vi "Robot_movimiento_calibración_NoLeeQR.vi"() -> ()   [LabVIEW 2019]
uses:
  <vilib>/Instr/_visa.llb/VISA Configure Serial Port (Instr).vi
  Global_STOP.vi
  <vilib>/regexp/Match Regular Expression.xnode
panel:
  in  "Bandeja Salida":bool=TRUE
  in  "stop socket 3":bool
  in  "stop 6":bool
  in  "Abrir socket 2":bool
  in  "Cerrar socket 2":bool
  in  "Interruptor Error 2":bool
  in  "stop 5":bool
  in  "STOP TEST 3":bool
  in  "Interruptor Error":bool
  in  "Cerrar socket":bool
  in  "Abrir socket":bool
  out "return count":u32
  out "lectura puerto serie":u32
  out "dato escrito puerto serie":string
  out "TEST OK":bool
  out "error out":errorcluster {"code" format="%f"}
  in  "STOP TEST 2":bool
  in  "SELECCION DE TEST":string(combo)="COMPLETO"
  in  "?":bool
  out "Boolean":bool
  in  "stop socket 2":bool
  out "Bytes at port 3":u32=1
  in  "IN y":string(combo)="00"
  in  "IN x":string(combo)="00"
  in  "NOK y":string(combo)="00"
  in  "NOK x":string(combo)="00"
  in  "OK y":string(combo)="00"
  in  "OK x":string(combo)="00"
  in  "Operator's name":string(combo)="Juan Rodríguez"
  in  "?":bool
  in  "Fichero de registro":path=path "C:/Trabajo_Robot/Pruebas/Pruebas.txt"
  in  "Path Out Report":path=path "C:/Trabajo_Robot/desde Marzo 2023/Pruebas_PC_APD/RESULT_TEST_C_LABP0/Test_33_ASIC_Referencia"
  in  "stop socket":bool
  out "Bytes at port 1":u32
  out "Iteraciones":i32
  out "Lectura buffer":string="1"
  in  "Delay (ms).Velocidad desplazamiento robot\nSi ponemos por ej. 2ms el robot va a la mitad de velocidad":dbl=1.0 min=1.0 max=9.0 step=1.0
  out "Bytes at port 2":u32=1
  in  "Interruptor":bool=TRUE
  in  "stop":bool
  # "SI SE PRESIONA EL BOTON STOP PARA INTERRUMPIR EL TEST,\nHAY QUE APAGAR Y VOLVER A ENCENDER EL ARDUINO\nCON EL SWITCH DE LA CAJA."
  # "TRUE : BANDEJA OK\nFALSE BANDEJA NOK"
  # "x: columna en cada bandeja \ny: fila en cada bandeja"
  # "Funcionamiento: en la primera iteración, el efector se desplaza desde el origen hasta la celda\nintroducida, hace una pausa, va a la posición del socket (0,0), hace otra pausa, va a la celda\nde salida y vuelve al origen. En las iteraciones siguientes hará lo mismo pero recorriendo las\nceldas de la bandeja sucesivamente. Que el desplazamiento se produzca hacia una celda de\nla bandeja OK o de la bandeja NOK depende de la salidad del programa de test de Asics."
types:
  T1 = enum16{"open", "replace", "create", "open or create", "replace or create", "replace or create with confirmation"}
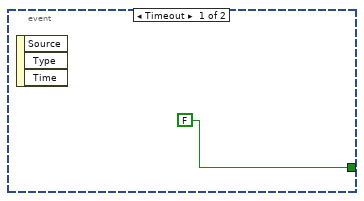
[diagram p2: hidden frame]
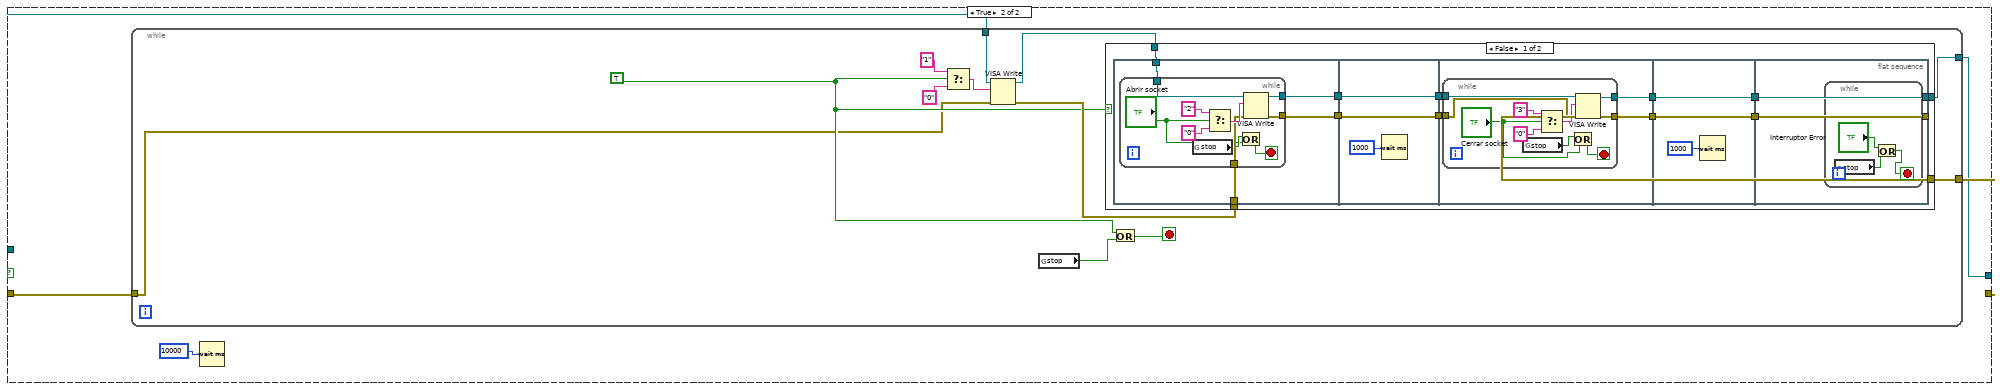
[diagram p3: hidden frame]
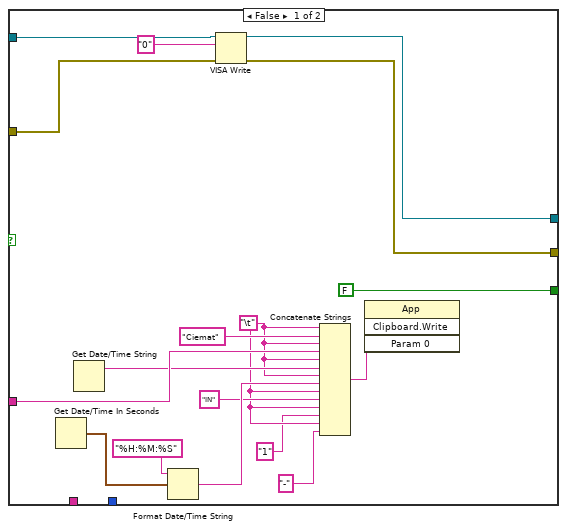
[diagram p5: hidden frame]
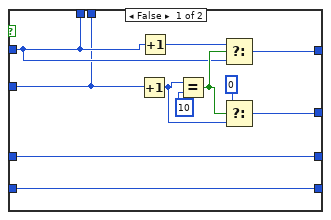
[diagram p7: hidden frame]
diagram:
  n1 = control-ref of="stop socket"() -> (w2:refnum<vi>)
  n2 = control-ref of="Cerrar socket"() -> (w10:refnum<vi>)
  n3 = control-ref of="STOP TEST 2"() -> (w13:refnum<vi>)
  n4 = control-ref of="Abrir socket"() -> (w8:refnum<vi>)
  n5 = control-ref of="stop"() -> (w9:refnum<vi>)
  n6 = control-ref of="Interruptor Error"() -> (w11:refnum<vi>)
  n7 = property class="Bool (strict)"(reference=w13, "Visible"=FALSE) -> ()  [unwired: 1 in, 2 out]
  n8 = property class="Bool"("Visible"=TRUE) -> ()  [unwired: 2 in, 2 out]
  n9 = property class="Bool (strict)"(reference=w8, "Visible"=FALSE) -> ()  [unwired: 1 in, 2 out]
  n10 = property class="Bool (strict)"(reference=w11, "Visible"=FALSE) -> ()  [unwired: 1 in, 2 out]
  n11 = property class="Bool (strict)"(reference=w10, "Visible"=FALSE) -> ()  [unwired: 1 in, 2 out]
  n12 = property on="Boolean" class="Bool (strict)"("Visible"=FALSE) -> ()  [unwired: 2 in, 2 out]
  n13 = property class="Bool"(reference=w2, "Visible"=FALSE) -> ()  [unwired: 1 in, 2 out]
  n14 = property class="Bool"(reference=w9, "Visible"=FALSE) -> ()  [unwired: 1 in, 2 out]
  n15 = flat-sequence {
    tunnel: [w56] -> w19
    tunnel: ["Fichero de registro"] -> w18
    tunnel: ["SELECCION DE TEST"] -> w17
    tunnel: ["NOK y"] -> w34
    tunnel: ["NOK x"] -> w33
    tunnel: ["OK y"] -> w32
    tunnel: ["OK x"] -> w31
    tunnel: ["IN y"] -> w30
    tunnel: ["IN x"] -> w29
    tunnel: [w59] -> w28
    tunnel: [w60] -> w27
    tunnel: ["IN y"] -> w26
    tunnel: ["IN x"] -> w25
    tunnel: w18 -> [w58]
    frame #0 {
      n16 = while {
        stop <- "?" stop-if-true
        n17 = Not(x="?") -> (.not. x?=w51:bool)
        "Boolean" <- w51
        n18 = property on="Boolean" class="Bool (strict)"("Blinking"=w51) -> ()  [unwired: 2 in, 2 out]
      }
      n19 = global write "Global_STOP.vi" "stop"(FALSE ("stop")) -> ()
    }
    frame #1 {
      n20 = property class="Bool"("Visible"=FALSE) -> ()  [unwired: 2 in, 2 out]
      n21 = Not(x="?") -> (.not. x?=w56:bool)
    }
    frame #2 {
      n22 = Open/Create/Replace File(file path (use dialog)=w58, operation (0:open)=T1."open", access (0:read/write)=enum16{"read/write", "read-only", "write-only"}."write-only") -> (refnum out=w71:refnum<file>, error out=w73:errorcluster)  [unwired: 3 in, 1 out]
      n23 = Set File Position(refnum=w71, from (0:start)=enum16{"start", "end", "current"}."end", error in=w73) -> (refnum out=w72:refnum<file>, error out=w74:errorcluster)  [unwired: 1 in]
      n24 = Write to Text File(file (use dialog)=w72, text="\r\n", error in=w74) -> (refnum out=w60:refnum<file>, error out=w59:errorcluster)  [unwired: 1 in, 1 out]
    }
  }
  n25 = Decimal String To Number(string=w26) -> (number=w24:i32)  [unwired: 2 in, 1 out]
  n26 = Decimal String To Number(string=w25) -> (number=w21:i32)  [unwired: 2 in, 1 out]
  n27 = Multiply(x=10, y=w24) -> (x*y=w22:i32)
  n28 = Decimal String To Number(string=w32) -> (number=w36:i32)  [unwired: 2 in, 1 out]
  n29 = Decimal String To Number(string=w31) -> (number=w35:i32)  [unwired: 2 in, 1 out]
  n30 = Decimal String To Number(string=w34) -> (number=w38:i32)  [unwired: 2 in, 1 out]
  n31 = Decimal String To Number(string=w33) -> (number=w37:i32)  [unwired: 2 in, 1 out]
  n32 = call-poly "VISA Configure Serial Port"("VISA resource name"=refnum<visa-resource-name> "COM9", "baud rate (9600)"=u32 9600, "data bits (8)"=u16 8) -> ("VISA resource name out"=w42:refnum<visa-resource-name>, "error out"=w45:errorcluster)  [unwired: 11 in]
  n33 = Add(x=w22, y=w21) -> (x+y=w20:i32)
  n34 = while {
    shift-right: [w75] -> w43
    shift-left: w45 -> [w116]
    tunnel: w42 -> [w114]
    tunnel: [w78] -> w44
    tunnel: w27 -> [w107]
    tunnel: [w106] -> w41
    tunnel: w28 -> [w105]
    tunnel: [w104] -> w40
    tunnel: w29 -> [w102]
    tunnel: w30 -> [w101]
    tunnel: w31 -> [w100]
    tunnel: w32 -> [w99]
    tunnel: w33 -> [w98]
    tunnel: w34 -> [w97]
    shift-right: [w90] -> _
    shift-left: w38 -> [w96]
    shift-right: [w92] -> _
    shift-left: w37 -> [w95]
    shift-right: [w89] -> _
    shift-left: w36 -> [w94]
    shift-right: [w91] -> _
    shift-left: w35 -> [w93]
    tunnel: w20 -> [w88]
    tunnel: w19 -> [w81]
    tunnel: w17 -> [w80]
    tunnel: [w77] -> w15
    i -> [w79]
    stop <- w77 stop-if-true
    # "Cuando Arduino deja un ASIC en la bandeja de  entrada ó en las de OK/NOK\ny vuelve a la posicion de socket, envia un \"2\" por el puerto serie\na labview y éste lo lee para que se salga del bucle, y prosiga la secuencia que le queda\nal programa, para después coger otro asic. Javier Morales"
    n35 = flat-sequence {
      tunnel: w116 -> [w154]
      tunnel: w114 -> [w143]
      tunnel: [w145] -> w113
      tunnel: [w144] -> w112
      tunnel: w102 -> [w124]
      tunnel: w101 -> [w123]
      tunnel: w100 -> [w122]
      tunnel: w99 -> [w121]
      tunnel: w98 -> [w120]
      tunnel: w97 -> [w119]
      tunnel: w113 -> [w891]
      tunnel: w112 -> [w890]
      tunnel: [w889] -> w87
      tunnel: [w888] -> w85
      tunnel: [w887] -> _
      tunnel: w87 -> [w908]
      tunnel: [w906] -> w86
      tunnel: w85 -> [w907]
      tunnel: [w905] -> w84
      tunnel: w86 -> [w928]
      tunnel: w84 -> [w927]
      tunnel: w79 -> [w929]
      tunnel: [w925] -> w83
      tunnel: [w924] -> w82
      tunnel: w79 -> [w1015]
      tunnel: [w1017] -> w110
      tunnel: [w1016] -> w109
      tunnel: [w1013] -> w103
      tunnel: w83 -> [w1012]
      tunnel: w82 -> [w1011]
      tunnel: w81 -> [w1006]
      tunnel: w80 -> [w1009]
      tunnel: w79 -> [w1008]
      tunnel: [w1065] -> w108
      tunnel: [w1067] -> w111
      tunnel: w110 -> [w1066]
      tunnel: w109 -> [w1064]
      tunnel: w107 -> [w1071]
      tunnel: [w1070] -> w106
      tunnel: w105 -> [w1069]
      tunnel: [w1068] -> w104
      tunnel: w79 -> [w1061]
      tunnel: w103 -> [w1060]
      tunnel: w96 -> [w1056]
      tunnel: w95 -> [w1059]
      tunnel: w94 -> [w1058]
      tunnel: w93 -> [w1057]
      tunnel: [w1055] -> w90
      tunnel: [w1054] -> w92
      tunnel: [w1053] -> w89
      tunnel: [w1052] -> w91
      tunnel: w88 -> [w1051]
      tunnel: w79 -> [w1050]
      tunnel: [w1049] -> _
      frame #0 {
        n36 = for {
          N: 2 -> [_]
          shift-right: [w766] -> _
          shift-left: w124 -> [w771]
          shift-right: [w769] -> w140
          shift-left: w143 -> [w770]
          shift-right: [w767] -> w139
          shift-left: w154 -> [w768]
          n37 = xnode "Match Regular Expression"("input string"=w771, "regular expression"="-?\\d") -> ("whole match"=w765:string, "after match"=w766:string)  [unwired: 4 in, 3 out]
          n38 = VISA Write(VISA resource name=w770, write buffer=w765, error in (no error)=w768) -> (VISA resource name out=w769:refnum<visa-resource-name>, error out=w767:errorcluster)  [unwired: 1 out]
        }
        n39 = for {
          N: 2 -> [_]
          shift-right: [w644] -> _
          shift-left: w123 -> [w649]
          shift-right: [w647] -> w134
          shift-left: w140 -> [w648]
          shift-right: [w645] -> w133
          shift-left: w139 -> [w646]
          n40 = xnode "Match Regular Expression"("input string"=w649, "regular expression"="-?\\d") -> ("whole match"=w643:string, "after match"=w644:string)  [unwired: 4 in, 3 out]
          n41 = VISA Write(VISA resource name=w648, write buffer=w643, error in (no error)=w646) -> (VISA resource name out=w647:refnum<visa-resource-name>, error out=w645:errorcluster)  [unwired: 1 out]
        }
        n42 = for {
          N: 2 -> [_]
          shift-right: [w522] -> _
          shift-left: w122 -> [w527]
          shift-right: [w525] -> w136
          shift-left: w134 -> [w526]
          shift-right: [w523] -> w135
          shift-left: w133 -> [w524]
          n43 = xnode "Match Regular Expression"("input string"=w527, "regular expression"="-?\\d") -> ("whole match"=w521:string, "after match"=w522:string)  [unwired: 4 in, 3 out]
          n44 = VISA Write(VISA resource name=w526, write buffer=w521, error in (no error)=w524) -> (VISA resource name out=w525:refnum<visa-resource-name>, error out=w523:errorcluster)  [unwired: 1 out]
        }
        n45 = for {
          N: 2 -> [_]
          shift-right: [w400] -> _
          shift-left: w121 -> [w405]
          shift-right: [w403] -> w128
          shift-left: w136 -> [w404]
          shift-right: [w401] -> w127
          shift-left: w135 -> [w402]
          n46 = xnode "Match Regular Expression"("input string"=w405, "regular expression"="-?\\d") -> ("whole match"=w399:string, "after match"=w400:string)  [unwired: 4 in, 3 out]
          n47 = VISA Write(VISA resource name=w404, write buffer=w399, error in (no error)=w402) -> (VISA resource name out=w403:refnum<visa-resource-name>, error out=w401:errorcluster)  [unwired: 1 out]
        }
        n48 = for {
          N: 2 -> [_]
          shift-right: [w278] -> _
          shift-left: w120 -> [w283]
          shift-right: [w281] -> w130
          shift-left: w128 -> [w282]
          shift-right: [w279] -> w129
          shift-left: w127 -> [w280]
          n49 = xnode "Match Regular Expression"("input string"=w283, "regular expression"="-?\\d") -> ("whole match"=w277:string, "after match"=w278:string)  [unwired: 4 in, 3 out]
          n50 = VISA Write(VISA resource name=w282, write buffer=w277, error in (no error)=w280) -> (VISA resource name out=w281:refnum<visa-resource-name>, error out=w279:errorcluster)  [unwired: 1 out]
        }
        n51 = for {
          N: 2 -> [_]
          shift-right: [w156] -> _
          shift-left: w119 -> [w161]
          shift-right: [w159] -> w126
          shift-left: w130 -> [w160]
          shift-right: [w157] -> w125
          shift-left: w129 -> [w158]
          n52 = xnode "Match Regular Expression"("input string"=w161, "regular expression"="-?\\d") -> ("whole match"=w155:string, "after match"=w156:string)  [unwired: 4 in, 3 out]
          n53 = VISA Write(VISA resource name=w160, write buffer=w155, error in (no error)=w158) -> (VISA resource name out=w159:refnum<visa-resource-name>, error out=w157:errorcluster)  [unwired: 1 out]
        }
        n54 = Number To Decimal String(number="Delay (ms).Velocidad desplazamiento robot\nSi ponemos por ej. 2ms el robot va a la mitad de velocidad") -> (decimal integer string=w148:string)  [unwired: 1 in]
        n55 = VISA Write(VISA resource name=w126, write buffer=w148, error in (no error)=w125) -> (VISA resource name out=w150:refnum<visa-resource-name>, error out=w149:errorcluster)  [unwired: 1 out]
        n56 = Select(t="1" ("write buffer"), s="Interruptor", f="0" ("write buffer")) -> (s? t:f=w146:string)
        n57 = VISA Write(VISA resource name=w150, write buffer=w146, error in (no error)=w149) -> (VISA resource name out=w145:refnum<visa-resource-name>, error out=w144:errorcluster)  [unwired: 1 out]
      }
      frame #1 {
        n58 = while {
          shift-right: [w898] -> w888
          shift-left: w890 -> [w903]
          tunnel: ["stop socket"] -> _
          shift-right: [w899] -> w889
          shift-left: w891 -> [w904]
          tunnel: ["stop socket"] -> w887
          stop <- w893 stop-if-true
          n59 = property class="Instr"(reference=w904, error in=w903) -> (reference out=w902:refnum<visa-resource-name>, error out=w901:errorcluster, "Bytes at Port"=w900:u32)
          "Bytes at port 1" <- w900
          n60 = VISA Read(VISA resource name=w902, byte count=w900, error in (no error)=w901) -> (VISA resource name out=w899:refnum<visa-resource-name>, read buffer=w897:string, error out=w898:errorcluster)  [unwired: 1 out]
          n61 = Equal?(x="2", y=w897) -> (x = y?=w895:bool)
          n62 = global read "Global_STOP.vi" "stop"() -> (w892:bool)
          n63 = Compound Arithmetic op=OR(w895, "stop socket", w892) -> (w893:bool)
        }
      }
      frame #2 {
        n64 = while {
          shift-right: [w915] -> w905
          shift-left: w907 -> [w920]
          tunnel: ["stop socket 2"] -> _
          shift-right: [w916] -> w906
          shift-left: w908 -> [w921]
          tunnel: ["stop socket 2"] -> _
          stop <- w910 stop-if-true
          n65 = property class="Instr"(reference=w921, error in=w920) -> (reference out=w919:refnum<visa-resource-name>, error out=w918:errorcluster, "Bytes at Port"=w917:u32)
          "Bytes at port 3" <- w917
          n66 = VISA Read(VISA resource name=w919, byte count=w917, error in (no error)=w918) -> (VISA resource name out=w916:refnum<visa-resource-name>, read buffer=w914:string, error out=w915:errorcluster)  [unwired: 1 out]
          n67 = Equal?(x="3", y=w914) -> (x = y?=w912:bool)
          n68 = global read "Global_STOP.vi" "stop"() -> (w909:bool)
          n69 = Compound Arithmetic op=OR(w912, "stop socket 2", w909) -> (w910:bool)
        }
      }
      frame #3 {
        # "Este bloque realiza la captura y lectura del QR"
        n70 = Greater?(x=w929, y=-1) -> (0:w926:bool)
        n71 = case shown="False" w926 {
          tunnel: [w932 w933] -> w924
          tunnel: w928 -> [w932 w935]
          tunnel: [w931 w934] -> w925
          tunnel: w927 -> [w931 w936]
          frame False {
          }
          frame True {
            n72 = while {
              tunnel: w935 -> [w949]
              tunnel: [w945] -> w933
              tunnel: [w944] -> w934
              tunnel: w936 -> [w938]
              stop <- w940 stop-if-true
              w939 = TRUE ("x")
              n73 = Select(t="1" ("write buffer"), s=w939, f="0" ("write buffer")) -> (s? t:f=w946:string)
              n74 = VISA Write(VISA resource name=w949, write buffer=w946, error in (no error)=w938) -> (VISA resource name out=w943:refnum<visa-resource-name>, error out=w942:errorcluster)  [unwired: 1 out]
              n75 = global read "Global_STOP.vi" "stop"() -> (w941:bool)
              n76 = case shown="False" w939 {
                tunnel: w943 -> [w961 w1002]
                tunnel: w942 -> [w960 w1001]
                tunnel: [w959 w1002] -> w945
                tunnel: [w958 w1001] -> w944
                frame False {
                  n77 = flat-sequence {
                    tunnel: w961 -> [w965]
                    tunnel: [w964] -> w957
                    tunnel: [w963] -> w955
                    tunnel: w960 -> [w962]
                    tunnel: w957 -> [w978]
                    tunnel: [w978] -> w956
                    tunnel: w955 -> [w977]
                    tunnel: [w977] -> w954
                    tunnel: w956 -> [w982]
                    tunnel: w954 -> [w981]
                    tunnel: [w980] -> w953
                    tunnel: [w979] -> w951
                    tunnel: w953 -> [w995]
                    tunnel: [w995] -> w952
                    tunnel: w951 -> [w994]
                    tunnel: [w994] -> w950
                    tunnel: [w996] -> w958
                    tunnel: [w997] -> w959
                    tunnel: w952 -> [w997]
                    tunnel: w950 -> [w996]
                    frame #0 {
                      n78 = while {
                        tunnel: w965 -> [w975]
                        tunnel: [w971] -> w964
                        tunnel: [w970] -> w963
                        tunnel: w962 -> [w969]
                        stop <- w966 stop-if-true
                        n79 = global read "Global_STOP.vi" "stop"() -> (w968:bool)
                        n80 = Select(t="2" ("write buffer"), s="Abrir socket", f="0" ("write buffer")) -> (s? t:f=w972:string)
                        n81 = Or(x=w968, y="Abrir socket") -> (x .or. y?=w966:bool)
                        n82 = VISA Write(VISA resource name=w975, write buffer=w972, error in (no error)=w969) -> (VISA resource name out=w971:refnum<visa-resource-name>, error out=w970:errorcluster)  [unwired: 1 out]
                      }
                    }
                    frame #1 {
                      n83 = Wait (ms)(milliseconds to wait=u32 1000) -> ()  [unwired: 1 out]
                    }
                    frame #2 {
                      n84 = while {
                        tunnel: w982 -> [w989]
                        tunnel: w981 -> [w988]
                        tunnel: [w987] -> w980
                        tunnel: [w986] -> w979
                        stop <- w985 stop-if-true
                        n85 = global read "Global_STOP.vi" "stop"() -> (w984:bool)
                        n86 = Select(t="3" ("write buffer"), s="Cerrar socket", f="0" ("write buffer")) -> (s? t:f=w990:string)
                        n87 = Or(x=w984, y="Cerrar socket") -> (x .or. y?=w985:bool)
                        n88 = VISA Write(VISA resource name=w989, write buffer=w990, error in (no error)=w988) -> (VISA resource name out=w987:refnum<visa-resource-name>, error out=w986:errorcluster)  [unwired: 1 out]
                      }
                    }
                    frame #3 {
                      n89 = Wait (ms)(milliseconds to wait=u32 1000) -> ()  [unwired: 1 out]
                    }
                    frame #4 {
                      n90 = while {
                        stop <- w998 stop-if-true
                        n91 = global read "Global_STOP.vi" "stop"() -> (w1000:bool)
                        n92 = Or(x="Interruptor Error", y=w1000) -> (x .or. y?=w998:bool)
                      }
                    }
                  }
                }
                frame True {
                }
              }
              n93 = Or(x=w939, y=w941) -> (x .or. y?=w940:bool)
            }
            n94 = Wait (ms)(milliseconds to wait=u32 10000) -> ()  [unwired: 1 out]
          }
        }
        n95 = control-ref of="STOP TEST 2"() -> (w923:refnum<vi>)
        n96 = property class="Bool (strict)"(reference=w923, "Visible"=TRUE) -> ()  [unwired: 1 in, 2 out]
      }
      frame #4 {
        n97 = global read "Global_STOP.vi" "stop"() -> (w1005:bool)
        n98 = Greater?(x=w1015, y=-1) -> (0:w1007:bool)
        n99 = Not(x=w1005) -> (.not. x?=w1004:bool)
        n100 = Compound Arithmetic op=AND(w1007, w1006, w1004) -> (w1003:bool)
        n101 = case shown="True" w1003 {
          tunnel: w1011 -> [w1032 w1040]
          tunnel: w1012 -> [w1031 w1039]
          tunnel: [w1030 w1038] -> w1017
          tunnel: [w1029 w1037] -> w1016
          tunnel: [FALSE ("Boolean") w1044] -> w1013
          tunnel: "Operator's name" -> [w1024 w1043]
          tunnel: w1009 -> [_ w1035]
          tunnel: w1008 -> [_ w1042]
          frame False {
            w1020 = "\t"
            n102 = Get Date/Time In Seconds() -> (seconds since 1Jan1904=w1027:timestamp)
            n103 = Get Date/Time String() -> (date string=w1023:string)  [unwired: 3 in, 1 out]
            n104 = Format Date/Time String(time format string (%c)="%H:%M:%S", seconds (now)=w1027) -> (date/time string=w1022:string)  [unwired: 1 in]
            n105 = VISA Write(VISA resource name=w1032, write buffer="0", error in (no error)=w1031) -> (VISA resource name out=w1030:refnum<visa-resource-name>, error out=w1029:errorcluster)  [unwired: 1 out]
            n106 = Concatenate Strings(w1020, "Ciemat", w1020, w1024, w1020, w1023, w1020, w1022, w1020, "IN", w1020, "1", w1020, "-") -> (w1028:string)
            n107 = invoke class="App" method="Clipboard.Write"("Param 0"=w1028) -> ()  [unwired: 3 in, 4 out]
          }
          frame True {
            # "Test de Asics"
            n108 = case shown="\"SOLO MOVIMIENTO\", Default" w1035 {
              tunnel: "Path Out Report" -> [_]
              tunnel: ["Bandeja Salida"] -> w1044
              tunnel: w1043 -> [_]
              tunnel: w1042 -> [_]
              frame "SOLO MOVIMIENTO", Default {
              }
            }
            "TEST OK" <- w1044
            n109 = Select(t="1" ("write buffer"), s=w1044, f="0" ("write buffer")) -> (s? t:f=w1041:string)
            "dato escrito puerto serie" <- w1041
            n110 = VISA Write(VISA resource name=w1040, write buffer=w1041, error in (no error)=w1039) -> (VISA resource name out=w1038:refnum<visa-resource-name>, return count=→"return count":u32, error out=w1037:errorcluster)
          }
        }
      }
      frame #5 {
        n111 = Greater?(x=w1061, y=-1) -> (0:w1062:bool)
        n112 = case shown="True" w1062 {
          tunnel: w1071 -> [w1077 w1110]
          tunnel: [w1077 w1109] -> w1070
          tunnel: w1069 -> [w1076 w1108]
          tunnel: [w1076 w1107] -> w1068
          tunnel: [w1079 w1106] -> w1067
          tunnel: w1066 -> [w1079 w1106]
          tunnel: [w1078 w1105] -> w1065
          tunnel: w1064 -> [w1078 w1105]
          tunnel: w1060 -> [_ w1103]
          tunnel: w1056 -> [w1075 w1102]
          tunnel: w1059 -> [w1074 w1101]
          tunnel: w1058 -> [w1073 w1100]
          tunnel: w1057 -> [w1072 w1099]
          tunnel: [w1075 w1098] -> w1055
          tunnel: [w1074 w1097] -> w1054
          tunnel: [w1073 w1096] -> w1053
          tunnel: [w1072 w1095] -> w1052
          frame False {
          }
          frame True {
            w1082 = "\t"
            # "Registro de datos en fichero"
            n113 = invoke class="App" method="Clipboard.Read"() -> ("Read Clipbrd"=w1104:string)  [unwired: 3 in, 2 out]
            n114 = case shown="True" w1103 {
              tunnel: w1102 -> [w1113 w1126]
              tunnel: w1101 -> [w1112 w1125]
              tunnel: w1100 -> [w1115 w1123]
              tunnel: w1099 -> [w1114 w1124]
              tunnel: [w1117 w1126] -> w1098
              tunnel: [w1116 w1125] -> w1097
              tunnel: [w1115 w1128] -> w1096
              tunnel: [w1114 w1127] -> w1095
              tunnel: [w1113 w1123] -> w1094
              tunnel: [w1112 w1124] -> w1093
              frame False {
                n115 = Increment(x=w1112) -> (x+1=w1121:i32)
                n116 = Increment(x=w1113) -> (x+1=w1118:i32)
                n117 = Equal?(x=w1121, y=10) -> (x = y?=w1119:bool)
                n118 = Select(t=w1118, s=w1119, f=w1113) -> (s? t:f=w1117:i32)
                n119 = Select(t=0, s=w1119, f=w1121) -> (s? t:f=w1116:i32)
              }
              frame True {
                n120 = Increment(x=w1124) -> (x+1=w1132:i32)
                n121 = Increment(x=w1123) -> (x+1=w1129:i32)
                n122 = Equal?(x=w1132, y=10) -> (x = y?=w1130:bool)
                n123 = Select(t=w1129, s=w1130, f=w1123) -> (s? t:f=w1128:i32)
                n124 = Select(t=0, s=w1130, f=w1132) -> (s? t:f=w1127:i32)
              }
            }
            n125 = Write to Text File(file (use dialog)=w1110, text=w1104, error in=w1108) -> (refnum out=w1091:refnum<file>, error out=w1092:errorcluster)  [unwired: 1 in, 1 out]
            n126 = Number To Decimal String(number=w1094) -> (decimal integer string=w1081:string)  [unwired: 1 in]
            n127 = Number To Decimal String(number=w1093) -> (decimal integer string=w1080:string)  [unwired: 1 in]
            n128 = Write to Text File(file (use dialog)=w1091, text=w1082, error in=w1092) -> (refnum out=w1089:refnum<file>, error out=w1090:errorcluster)  [unwired: 1 in, 1 out]
            n129 = Write to Text File(file (use dialog)=w1089, text=w1081, error in=w1090) -> (refnum out=w1086:refnum<file>, error out=w1085:errorcluster)  [unwired: 1 in, 1 out]
            n130 = Write to Text File(file (use dialog)=w1086, text=w1082, error in=w1085) -> (refnum out=w1084:refnum<file>, error out=w1083:errorcluster)  [unwired: 1 in, 1 out]
            n131 = Write to Text File(file (use dialog)=w1084, text=w1080, error in=w1083) -> (refnum out=w1088:refnum<file>, error out=w1087:errorcluster)  [unwired: 1 in, 1 out]
            n132 = Write to Text File(file (use dialog)=w1088, text="\r\n", error in=w1087) -> (refnum out=w1109:refnum<file>, error out=w1107:errorcluster)  [unwired: 1 in, 1 out]
          }
        }
        n133 = Add(x=w1051, y=w1050) -> (x+y=w1049:i32)
      }
    }
    n134 = while {
      shift-right: [w1141] -> w76
      shift-left: w108 -> [w1147]
      tunnel: ["stop"] -> _
      shift-right: [w1142] -> w78
      shift-left: w111 -> [w1148]
      tunnel: [w1137] -> w115
      stop <- w1135 stop-if-true
      # "1"
      n135 = property class="Instr"(reference=w1148, error in=w1147) -> (reference out=w1145:refnum<visa-resource-name>, error out=w1144:errorcluster, "Bytes at Port"=w1143:u32)
      "Bytes at port 2" <- w1143
      n136 = VISA Read(VISA resource name=w1145, byte count=w1143, error in (no error)=w1144) -> (VISA resource name out=w1142:refnum<visa-resource-name>, read buffer=w1137:string, return count=w1140:u32, error out=w1141:errorcluster)
      "lectura puerto serie" <- w1140
      n137 = Greater Or Equal?(x=w1140, y=u32 1) -> (x >= y?=w1138:bool)
      n138 = global read "Global_STOP.vi" "stop"() -> (w1134:bool)
      n139 = Or(x=w1138, y="stop") -> (x .or. y?=w1136:bool)
      n140 = Compound Arithmetic op=OR(w1136, w1134) -> (w1135:bool)
    }
    "Lectura buffer" <- w115
    n141 = flat-sequence {
      tunnel: [w117] -> w77
      tunnel: [w118] -> w75
      tunnel: w76 -> [w118]
      frame #0 {
        n142 = global read "Global_STOP.vi" "stop"() -> (w117:bool)
      }
    }
    "Iteraciones" <- w79
  }
  n143 = flat-sequence {
    frame #0 {
      n144 = local write "STOP TEST 2"(FALSE ("STOP TEST 2")) -> ()
    }
    frame #1 {
      n145 = while {
        stop <- w1150 stop-if-true
        n146 = event shown="[1] \"STOP TEST 2\": Value Change" {
          selector: _ -> [_ _]
          dyn-events: _ -> [_ _]
          timeout: _ -> [_ _]
          tunnel: [FALSE "STOP TEST 2"] -> w1150
          event Timeout {
            n147 = event-data() -> ()  [unwired: 1 in, 3 out]
          }
          event "STOP TEST 2": Value Change {
            n148 = event-data() -> ()  [unwired: 1 in, 6 out]
            n149 = global write "Global_STOP.vi" "stop"("STOP TEST 2") -> ()
            n150 = Wait (ms)(milliseconds to wait=u32 100) -> ()  [unwired: 1 out]
          }
        }
      }
    }
  }
  n151 = Close File(refnum=w41, error in=w40) -> (error out=w39:errorcluster)  [unwired: 1 out]
  n152 = Not(x=w15) -> (.not. x?=w16:bool)
  n153 = call <vilib>:"Simple Error Handler.vi"("error in (no error)"=w39) -> ()  [unwired: 4 in, 5 out]
  n154 = global write "Global_STOP.vi" "stop"(w16) -> ()
  n155 = VISA Close(VISA resource name=w44, error in (no error)=w43) -> (error out=→"error out":errorcluster)
